vi "Send Parameter.vi"(8 "error in (no error)":errorcluster, 10 "Value":refnum<class>, 11 "Future in":refnum<class "Future.lvclass">) -> (0 "error out":errorcluster, 3 "Future out":refnum<class "Future.lvclass">)   [LabVIEW 2020, in "Promises.lvlib" / "Future.lvclass"]
doc: "Sends an input parameter through the Promise. Sending an input parameter is task dependent; not every task will be implemented to require a parameter input to begin work.\n\nThis VI will generate an error if a parameter has already been sent in the promise."
uses:
  Future.lvclass
  Error Result/Error Result.lvclass
  Error Result/Error Result.lvclass/Error Result.ctl
  Future.lvclass/Future.ctl
  Parameter Data.ctl
  Promises.lvlib
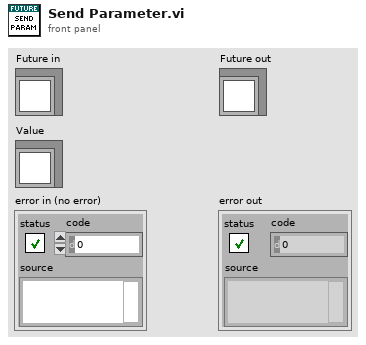
[diagram p1: front panel]
types:
  T1 = typedef "Promises.lvlib/Parameter Data.ctl" = cluster{"Parameter":refnum<class>}
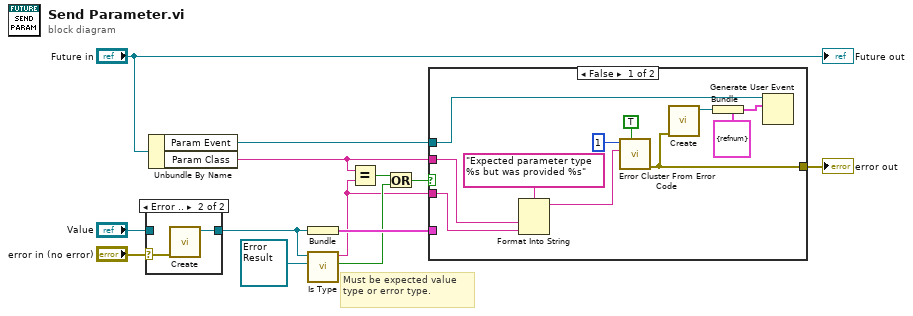
[diagram p0: block diagram]
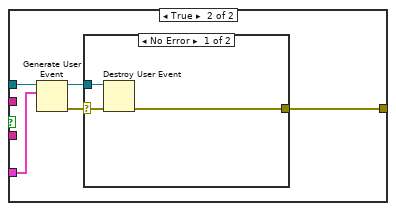
[diagram p3: hidden frame]
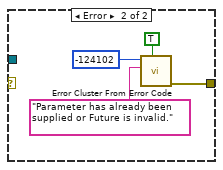
[diagram p4: hidden frame]
diagram:
  # "Must be expected value type or error type."
  n1 = case shown="Error .." "error in (no error)" {
    selector: "error in (no error)" -> [_ w16]
    tunnel: "Value" -> [w14 _]
    tunnel: [w14 w15] -> w7
    frame No Error {
    }
    frame Error {
      n2 = call "Create.vi"("error in (no error)"=w16) -> ("Error Result out"=w15:refnum<class "Error Result.lvclass">)  [unwired: 9 in, 1 out]
    }
  }
  n3 = Unbundle By Name("Future in") -> ("Param Event"=w11:refnum<user-event>, "Param Class"=w13:string)
  n4 = Bundle("Value"=w7) -> (w10:cluster{"Value":refnum<class>})  [unwired: 1 in]
  n5 = call "Is Type.vi"("Type"=refnum<class "Error Result.lvclass"> refnum ("Futures:Error Result.lvclass"), "Value"=w7) -> ("Type Matches"=w2:bool, "Value Class"=w1:string)  [unwired: 8 in]
  n6 = Equal?(x=w13, y=w1) -> (x = y?=w12:bool)
  n7 = Or(x=w12, y=w2) -> (x .or. y?=w8:bool)
  n8 = case shown="False" w8 {
    tunnel: w10 -> [_ w28]
    tunnel: w13 -> [w27 _]
    tunnel: w1 -> [w26 _]
    tunnel: w11 -> [w20 w32]
    tunnel: [w21 w29] -> w3
    frame False {
      n9 = Format Into String(format string="Expected parameter type %s but was provided %s", w27, w26) -> (resulting string=w23:string)  [unwired: 2 in, 1 out]
      n10 = call <vilib>:"Error Cluster From Error Code.vi"("show call chain? (False)"=TRUE, "error message (\"\")"=w23, "error code (0)"=1) -> ("error out"=w21:errorcluster)  [unwired: 6 in]
      n11 = call "Create.vi"("error in (no error)"=w21) -> ("Error Result out"=w19:refnum<class "Error Result.lvclass">)  [unwired: 9 in, 1 out]
      n12 = Bundle(cluster=T1 {"Parameter"=refnum} ("Parameter Data"), "Parameter"=w19) -> (w18:T1)
      n13 = Generate User Event(user event=w20, event data cluster=w18) -> ()  [unwired: 2 in, 2 out]
    }
    frame True {
      n14 = Generate User Event(user event=w32, event data cluster=w28) -> (user event out=w30:refnum<user-event>, error out=w31:errorcluster)  [unwired: 2 in]
      n15 = case shown="No Error" w31 {
        selector: w31 -> [w34 _]
        tunnel: w30 -> [w35 _]
        tunnel: [w33 w39] -> w29
        frame No Error {
          n16 = Destroy User Event(user event=w35, error in=w34) -> (error out=w33:errorcluster)
        }
        frame Error {
          n17 = call <vilib>:"Error Cluster From Error Code.vi"("show call chain? (False)"=TRUE, "error message (\"\")"="Parameter has already been supplied or Future is invalid.", "error code (0)"=-124102) -> ("error out"=w39:errorcluster)  [unwired: 6 in]
        }
      }
    }
  }
  "error out" <- w3
  "Future out" <- "Future in"
